vi "4.2.vi"() -> ()   [LabVIEW 2017]
panel:
  in  "停止":bool
  out "波形图表":cluster{"number: 0 to 1":dbl, dbl, dbl}(graph)
  # "任务一"
  # "任务二"
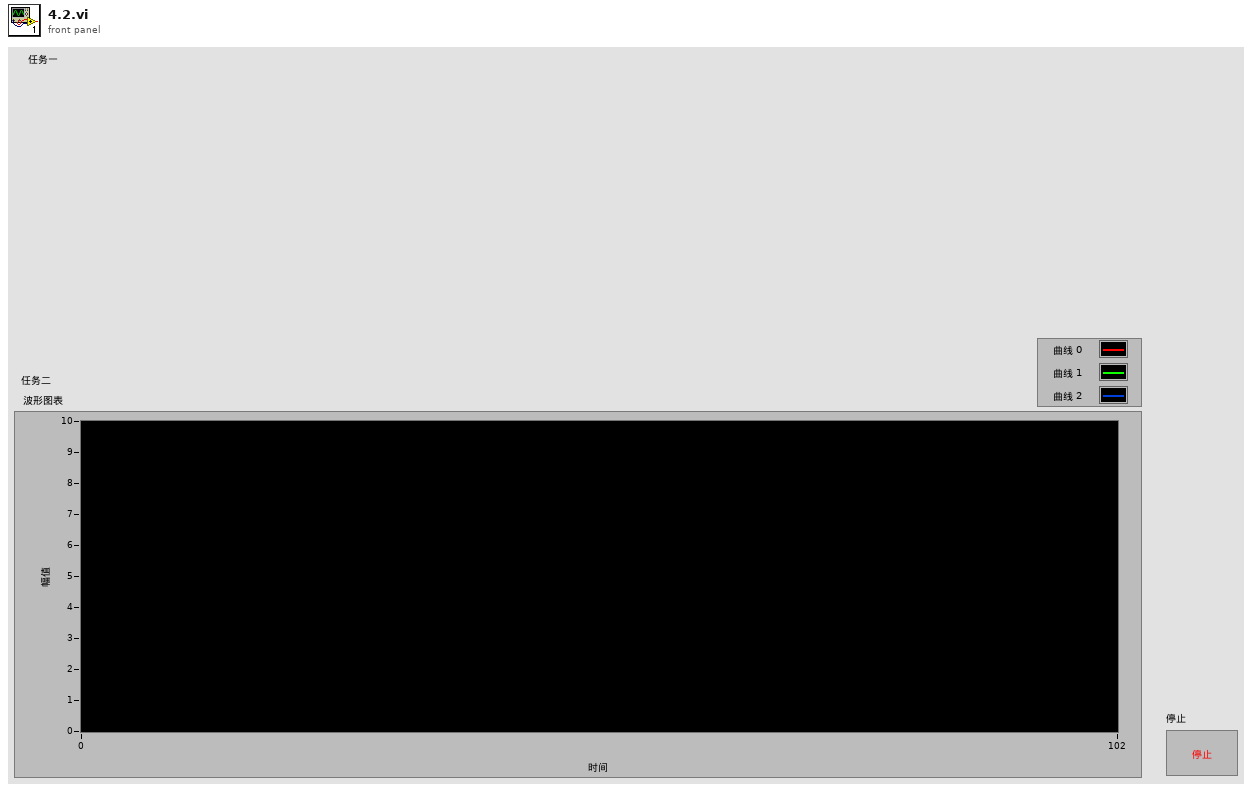
[diagram p1: front panel]
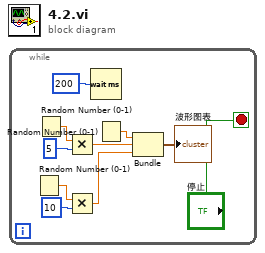
[diagram p0: block diagram]
diagram:
  n1 = while {
    stop <- "停止" stop-if-true
    n2 = Random Number (0-1)() -> (number: 0 to 1=w7:dbl)
    n3 = Random Number (0-1)() -> (number: 0 to 1=w8:dbl)
    n4 = Multiply(x=w8, y=5) -> (x*y=w5:dbl)
    n5 = Multiply(x=w7, y=10) -> (x*y=w4:dbl)
    n6 = Wait (ms)(milliseconds to wait=200) -> ()  [unwired: 1 out]
    n7 = Random Number (0-1)() -> (number: 0 to 1=w6:dbl)
    n8 = Bundle("number: 0 to 1"=w6, w5, w4) -> (→"波形图表":cluster{"number: 0 to 1":dbl, dbl, dbl})  [unwired: 1 in]
  }
